vi "Run_preset_commands.vi"() -> ()   [LabVIEW 2022 SP3]
uses:
  Command_buttons.ctl
  ctl_timer_fgv_states_enum.ctl
  Prog_time_control.ctl
  Written_command.ctl
panel:
  out "Command to write":T1
  in  "Temp1 reached?":bool
  in  "Temperature-time program":T2
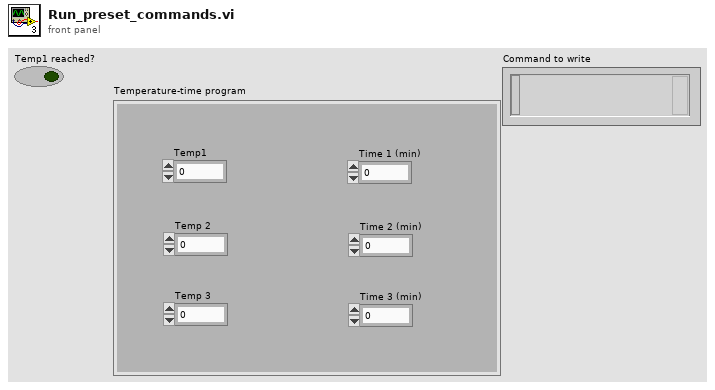
[diagram p1: front panel]
types:
  T1 = typedef "Written_command.ctl" = string
  T2 = typedef "Prog_time_control.ctl" = cluster{"Temp1":dbl, "Temp 2":dbl, "Temp 3":dbl, "Time 1 (min)":dbl, "Time 2 (min)":dbl, "Time 3 (min)":dbl}
  T3 = typedef "Command_buttons.ctl" = enum32{"P0", "P1", "F?", "S?", "Sn", "UC", "UF"}
  T4 = typedef "ctl_timer_fgv_states_enum.ctl" = enum16{"RESET", "GET"}
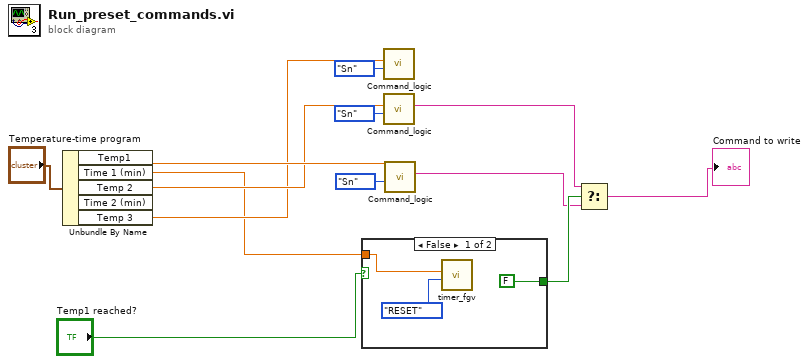
[diagram p0: block diagram]
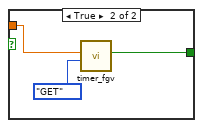
[diagram p2: hidden frame]
diagram:
  n1 = Unbundle By Name("Temperature-time program") -> ("Temp1"=w11:dbl, "Time 1 (min)"=w2:dbl, "Temp 2"=w6:dbl, "Temp 3"=w4:dbl)  [unwired: 1 out]
  n2 = case shown="False" "Temp1 reached?" {
    tunnel: [FALSE ("TIme passed?") w18] -> w10
    tunnel: w2 -> [w14 w17]
    frame False {
      n3 = call "timer_fgv.vi"("Operation"=ctl_timer_fgv_states_enum."RESET", "TImer"=w14) -> ()  [unwired: 9 in, 1 out]
    }
    frame True {
      n4 = call "timer_fgv.vi"("Operation"=ctl_timer_fgv_states_enum."GET", "TImer"=w17) -> ("TIme passed?"=w18:bool)  [unwired: 9 in]
    }
  }
  n5 = call "Command_logic.vi"("Command Radio Buttons"=Command_buttons."Sn", "Temperature\nto set"=w4) -> ()  [unwired: 9 in, 1 out]
  n6 = call "Command_logic.vi"("Command Radio Buttons"=Command_buttons."Sn", "Temperature\nto set"=w6) -> ("Written command"=w7:T1)  [unwired: 9 in]
  n7 = call "Command_logic.vi"("Command Radio Buttons"=Command_buttons."Sn", "Temperature\nto set"=w11) -> ("Written command"=w9:T1)  [unwired: 9 in]
  n8 = Select(t=w7, s=w10, f=w9) -> (s? t:f=→"Command to write":T1)
